vi "Motors Move Absolute.vi"(5 "Axis Multiplier":u32, 7 "Axis":u32=1, 8 "error in":errorcluster, 9 "VISA in":refnum<visa-resource-name>, 11 "Position (mm or degree)":dbl) -> (0 "error out":errorcluster, 1 "VISA out":refnum<visa-resource-name>)   [LabVIEW 2018]
panel:
  out "Read Buffer":string
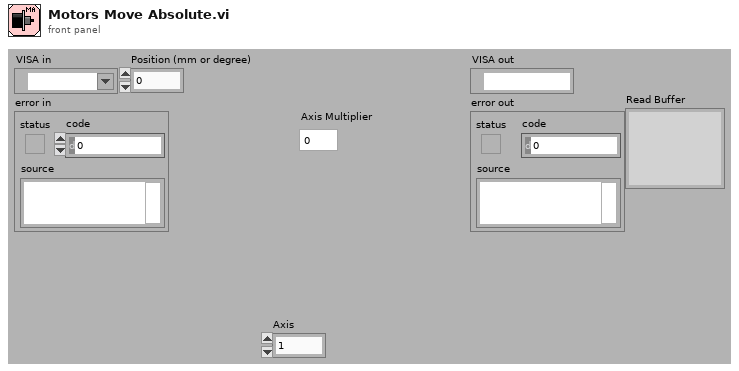
[diagram p1: front panel]
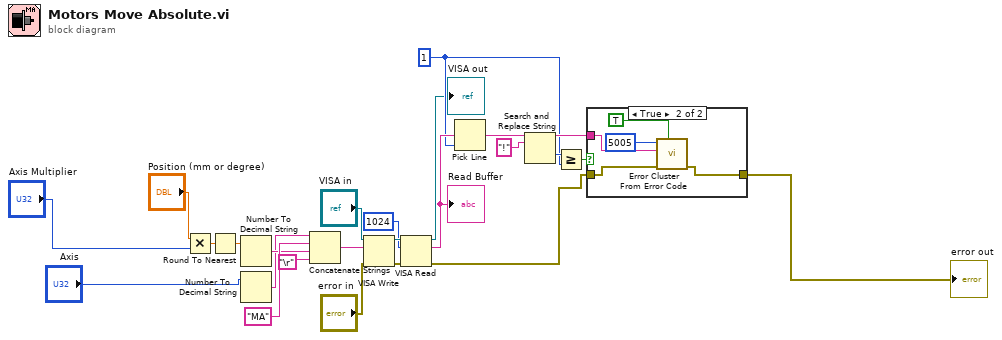
[diagram p0: block diagram]
diagram:
  w12 = 1 ("line index")
  n1 = Multiply(x="Position (mm or degree)", y="Axis Multiplier") -> (x*y=w5:dbl)
  n2 = Round To Nearest(number=w5) -> (nearest integer value=w4:dbl)
  n3 = Number To Decimal String(number=w4) -> (decimal integer string=w24:string)  [unwired: 1 in]
  n4 = Number To Decimal String(number="Axis") -> (decimal integer string=w15:string)  [unwired: 1 in]
  n5 = Concatenate Strings(w15, "MA", w24, "\r") -> (w9:string)
  n6 = VISA Write(VISA resource name="VISA in", write buffer=w9, error in (no error)="error in") -> (VISA resource name out=w23:refnum<visa-resource-name>, error out=w22:errorcluster)  [unwired: 1 out]
  n7 = VISA Read(VISA resource name=w23, byte count=1024, error in (no error)=w22) -> (VISA resource name out=→"VISA out":refnum<visa-resource-name>, read buffer=w19:string, error out=w1:errorcluster)  [unwired: 1 out]
  "Read Buffer" <- w19
  n8 = Pick Line(multi-line string=w19, line index=w12) -> (output string=w21:string)  [unwired: 1 in]
  n9 = Search and Replace String(input string=w21, search string="!") -> (result string=w16:string, offset past replacement=w18:i32)  [unwired: 6 in, 2 out]
  n10 = Greater Or Equal?(x=w18, y=w12) -> (x >= y?=w17:bool)
  n11 = case shown="True" w17 {
    tunnel: w16 -> [_ w29]
    tunnel: [w26 w30] -> w2
    tunnel: w1 -> [w26 w31]
    frame False {
    }
    frame True {
      n12 = call <vilib>:"Error Cluster From Error Code.vi"("show call chain? (False)"=TRUE, "error in (no error)"=w31, "error message (\"\")"=w29, "error code (0)"=5005) -> ("error out"=w30:errorcluster)  [unwired: 5 in]
    }
  }
  "error out" <- w2
